vi "pick 2 ball.vi"   [LabVIEW 2016, in "Test2.lvrbt"]
uses:
  Test2.lvrbt
  <vilib>/NXT/Hardware/Plugins/Tetrix 180 deg Servo/Tetrix180ServoAddress.ctl
  <vilib>/NXT/Hardware/Plugins/Tetrix DC Motor/TetrixDCMotorAddress.ctl
  <vilib>/NXT/Block Support/NXT_InputPort.ctl
  <vilib>/NXT/NXTIO Xnodes/NXTIONodeSubVIs/TETRIX IO Move Servos.vi
  <vilib>/NXT/Dual Mode Library/Waits/Wait_Num.vi
  <vilib>/NXT/NXTIO Xnodes/NXTIONodeSubVIs/TETRIX IO Move DC Motors.vi
  <vilib>/NXT/Dual Mode Library/Waits/Wait_EV3_Ultrasonic_Centimeters_Further.vi
  <vilib>/NXT/NXTIO Xnodes/NXTIONodeSubVIs/TETRIX IO Stop DC Motors.vi
  <vilib>/NXT/Dual Mode Library/Waits/Wait_EV3_Ultrasonic_Centimeter_Closer.vi
  <vilib>/NXT/Subs/LVHSConnector.ctl
  <vilib>/NXT/NXTIO Xnodes/AddressXNode/NXTIOAddress.xnode
  <vilib>/NXT/NXTIO Xnodes/NXTIOXNode/NXTIO.xnode
  <vilib>/NXT/LegoClasses/BrickReference/BrickReference.lvclass
types:
  T1 = typedef "Tetrix180ServoAddress.ctl" = i32
  T2 = cluster{"Tetrix180Servo":T1, "Tetrix180Servo":T1, "Tetrix180Servo":T1, "Tetrix180Servo":T1, "Tetrix180Servo":T1, "Tetrix180Servo":T1}
  T3 = typedef "LVHSConnector.ctl" = refnum<class "BrickReference.lvclass">
  T4 = typedef "TetrixDCMotorAddress.ctl" = i32
  T5 = typedef "NXT_InputPort.ctl" = u32
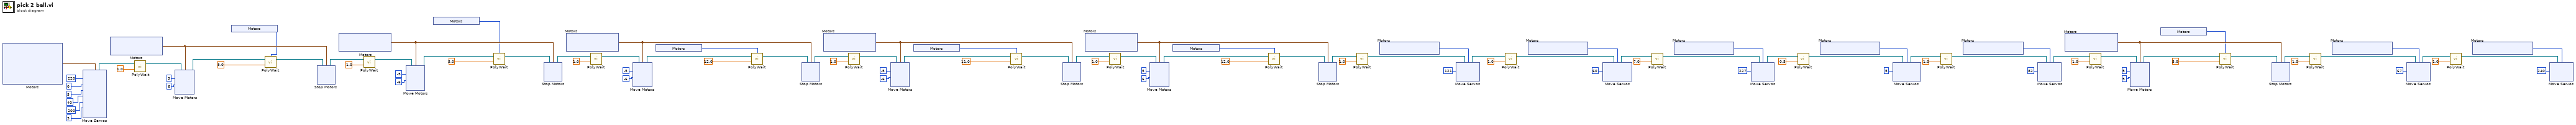
[diagram p0: block diagram]
diagram:
  n1 = xnode "Motors"() -> ("Motor"=w102:T2)
  n2 = xnode "Move Servos"("Position 6"=u8 5, "Position 5"=u8 200, "Position 4"=u8 40, "Position 3"=u8 5, "Position 2"=u8 0, "Position 1"=u8 220, "Motors"=w102) -> ("NXT/EV3"=w80:T3)  [unwired: 1 in]
  n3 = xnode "Motors"() -> ("Motor"=w91:cluster{"TetrixDCMotor":T4, "TetrixDCMotor":T4})
  n4 = call-poly <vilib>:"PolyWait.vi"("Time (1 sec)"=sgl 1.0, "NXT/EV3"=w80) -> ("NXT/EV3"=w79:T3)  [unwired: 2 in]
  n5 = xnode "Move Motors"("Power/Speed 2"=i8 6, "Power/Speed 1"=i8 5, "Motors"=w91, "NXT/EV3"=w79) -> ("NXT/EV3"=w94:T3)
  n6 = xnode "Motors"() -> ("Sensor"=w3:T5)
  n7 = call-poly <vilib>:"PolyWait.vi"("Centimeters (50)"=sgl 5.0, "NXT/EV3"=w94, "Port (Port 1)"=w3) -> ("NXT/EV3"=w92:T3)  [unwired: 1 in]
  n8 = xnode "Stop Motors"("Motors"=w91, "NXT/EV3"=w92) -> ("NXT/EV3"=w78:T3)
  n9 = xnode "Motors"() -> ("Motor"=w71:cluster{"TetrixDCMotor":T4, "TetrixDCMotor":T4})
  n10 = call-poly <vilib>:"PolyWait.vi"("Time (1 sec)"=sgl 1.0, "NXT/EV3"=w78) -> ("NXT/EV3"=w10:T3)  [unwired: 2 in]
  n11 = xnode "Move Motors"("Power/Speed 2"=i8 -6, "Power/Speed 1"=i8 -5, "Motors"=w71, "NXT/EV3"=w10) -> ("NXT/EV3"=w73:T3)
  n12 = xnode "Motors"() -> ("Sensor"=w2:T5)
  n13 = call-poly <vilib>:"PolyWait.vi"("Centimeters (40)"=sgl 5.0 ("Centimeters (50)"), "NXT/EV3"=w73, "Port (Port 1)"=w2) -> ("NXT/EV3"=w72:T3)  [unwired: 1 in]
  n14 = xnode "Stop Motors"("Motors"=w71, "NXT/EV3"=w72) -> ("NXT/EV3"=w70:T3)
  n15 = xnode "Motors"() -> ("Motor"=w84:cluster{"TetrixDCMotor":T4, "TetrixDCMotor":T4})
  n16 = call-poly <vilib>:"PolyWait.vi"("Time (1 sec)"=sgl 1.0, "NXT/EV3"=w70) -> ("NXT/EV3"=w87:T3)  [unwired: 2 in]
  n17 = xnode "Move Motors"("Power/Speed 2"=i8 -6, "Power/Speed 1"=i8 -5, "Motors"=w84, "NXT/EV3"=w87) -> ("NXT/EV3"=w86:T3)
  n18 = xnode "Motors"() -> ("Sensor"=w82:T5)
  n19 = call-poly <vilib>:"PolyWait.vi"("Centimeters (40)"=sgl 12.0 ("Centimeters (50)"), "NXT/EV3"=w86, "Port (Port 1)"=w82) -> ("NXT/EV3"=w85:T3)  [unwired: 1 in]
  n20 = xnode "Stop Motors"("Motors"=w84, "NXT/EV3"=w85) -> ("NXT/EV3"=w62:T3)
  n21 = xnode "Motors"() -> ("Motor"=w61:cluster{"TetrixDCMotor":T4, "TetrixDCMotor":T4})
  n22 = call-poly <vilib>:"PolyWait.vi"("Time (1 sec)"=sgl 1.0, "NXT/EV3"=w62) -> ("NXT/EV3"=w67:T3)  [unwired: 2 in]
  n23 = xnode "Move Motors"("Power/Speed 2"=i8 -6, "Power/Speed 1"=i8 -5, "Motors"=w61, "NXT/EV3"=w67) -> ("NXT/EV3"=w66:T3)
  n24 = xnode "Motors"() -> ("Sensor"=w63:T5)
  n25 = call-poly <vilib>:"PolyWait.vi"("Centimeters (50)"=sgl 11.0, "NXT/EV3"=w66, "Port (Port 1)"=w63) -> ("NXT/EV3"=w65:T3)  [unwired: 1 in]
  n26 = xnode "Stop Motors"("Motors"=w61, "NXT/EV3"=w65) -> ("NXT/EV3"=w12:T3)
  n27 = xnode "Motors"() -> ("Motor"=w15:cluster{"TetrixDCMotor":T4, "TetrixDCMotor":T4})
  n28 = call-poly <vilib>:"PolyWait.vi"("Time (1 sec)"=sgl 1.0, "NXT/EV3"=w12) -> ("NXT/EV3"=w18:T3)  [unwired: 2 in]
  n29 = xnode "Move Motors"("Power/Speed 2"=i8 6, "Power/Speed 1"=i8 5, "Motors"=w15, "NXT/EV3"=w18) -> ("NXT/EV3"=w17:T3)
  n30 = xnode "Motors"() -> ("Sensor"=w13:T5)
  n31 = call-poly <vilib>:"PolyWait.vi"("Centimeters (40)"=sgl 12.0 ("Centimeters (50)"), "NXT/EV3"=w17, "Port (Port 1)"=w13) -> ("NXT/EV3"=w16:T3)  [unwired: 1 in]
  n32 = xnode "Stop Motors"("Motors"=w15, "NXT/EV3"=w16) -> ("NXT/EV3"=w5:T3)
  n33 = call-poly <vilib>:"PolyWait.vi"("Time (1 sec)"=sgl 1.0, "NXT/EV3"=w5) -> ("NXT/EV3"=w7:T3)  [unwired: 2 in]
  n34 = xnode "Motors"() -> ("Motor"=w6:T1)
  n35 = xnode "Move Servos"("Position 1"=u8 121, "Motors"=w6, "NXT/EV3"=w7) -> ("NXT/EV3"=w4:T3)
  n36 = call-poly <vilib>:"PolyWait.vi"("Time (1 sec)"=sgl 1.0, "NXT/EV3"=w4) -> ("NXT/EV3"=w33:T3)  [unwired: 2 in]
  n37 = xnode "Motors"() -> ("Motor"=w52:T1)
  n38 = xnode "Move Servos"("Position 1"=u8 60, "Motors"=w52, "NXT/EV3"=w33) -> ("NXT/EV3"=w49:T3)
  n39 = call-poly <vilib>:"PolyWait.vi"("Time (1 sec)"=sgl 7.0, "NXT/EV3"=w49) -> ("NXT/EV3"=w46:T3)  [unwired: 2 in]
  n40 = xnode "Motors"() -> ("Motor"=w48:T1)
  n41 = xnode "Move Servos"("Position 1"=u8 227, "Motors"=w48, "NXT/EV3"=w46) -> ("NXT/EV3"=w44:T3)
  n42 = call-poly <vilib>:"PolyWait.vi"("Time (1 sec)"=sgl 0.5, "NXT/EV3"=w44) -> ("NXT/EV3"=w41:T3)  [unwired: 2 in]
  n43 = xnode "Motors"() -> ("Motor"=w43:T1)
  n44 = xnode "Move Servos"("Position 1"=u8 5, "Motors"=w43, "NXT/EV3"=w41) -> ("NXT/EV3"=w39:T3)
  n45 = call-poly <vilib>:"PolyWait.vi"("Time (1 sec)"=sgl 1.0, "NXT/EV3"=w39) -> ("NXT/EV3"=w36:T3)  [unwired: 2 in]
  n46 = xnode "Motors"() -> ("Motor"=w37:T1)
  n47 = xnode "Move Servos"("Position 1"=u8 82, "Motors"=w37, "NXT/EV3"=w36) -> ("NXT/EV3"=w35:T3)
  n48 = xnode "Motors"() -> ("Motor"=w55:cluster{"TetrixDCMotor":T4, "TetrixDCMotor":T4})
  n49 = call-poly <vilib>:"PolyWait.vi"("Time (1 sec)"=sgl 1.0, "NXT/EV3"=w35) -> ("NXT/EV3"=w53:T3)  [unwired: 2 in]
  n50 = xnode "Move Motors"("Power/Speed 2"=i8 5, "Power/Speed 1"=i8 5, "Motors"=w55, "NXT/EV3"=w53) -> ("NXT/EV3"=w57:T3)
  n51 = xnode "Motors"() -> ("Sensor"=w1:T5)
  n52 = call-poly <vilib>:"PolyWait.vi"("Centimeters (50)"=sgl 5.0, "NXT/EV3"=w57, "Port (Port 1)"=w1) -> ("NXT/EV3"=w56:T3)  [unwired: 1 in]
  n53 = xnode "Stop Motors"("Motors"=w55, "NXT/EV3"=w56) -> ("NXT/EV3"=w30:T3)
  n54 = call-poly <vilib>:"PolyWait.vi"("Time (1 sec)"=sgl 1.0, "NXT/EV3"=w30) -> ("NXT/EV3"=w27:T3)  [unwired: 2 in]
  n55 = xnode "Motors"() -> ("Motor"=w28:T1)
  n56 = xnode "Move Servos"("Position 1"=u8 67, "Motors"=w28, "NXT/EV3"=w27) -> ("NXT/EV3"=w25:T3)
  n57 = call-poly <vilib>:"PolyWait.vi"("Time (1 sec)"=sgl 1.0, "NXT/EV3"=w25) -> ("NXT/EV3"=w22:T3)  [unwired: 2 in]
  n58 = xnode "Motors"() -> ("Motor"=w23:T1)
  n59 = xnode "Move Servos"("Position 1"=u8 240, "Motors"=w23, "NXT/EV3"=w22) -> ()  [unwired: 1 out]
